vi "Initialize Global Log.vi"(6 "iName":string, 7 "Configuration.Level":T1=enum."Debug", 8 "error in (no error)":errorcluster, 11 "Mediated Actor in":refnum<class "Mediated Actor.lvclass">) -> (0 "error out":errorcluster, 3 "Mediated Actor out":refnum<class "Mediated Actor.lvclass">)   [LabVIEW 2016, in "Stream Mediator.lvlib" / "Mediated Actor.lvclass"]
doc: "--\nCopyright © 2017 Composed SystemsI All rights reserved.\n\nAuthor: Jon McBee <jon.mcbee@composed.io>\n\nThis library is provided \"AS IS\" ,WITHOUT WARRANTIES OR\nCONDITIONS OF ANY KIND, either express or implied.\n\nComposed Systems -- composed.io\n\nStream 0.0.1.1\nJon McBee - Composed Systems\nCopyright (c) 2017, Composed Systems"
uses:
  <userlib>/Composed Systems/Stream/Mediator/Classes/Mediated Actor/Mediated Actor.lvclass
  <userlib>/Composed Systems/Stream/Log/Application Log/Log Level.ctl
  <userlib>/Composed Systems/Stream/Log/Asynchronous Application Log/Asynchronous Application Log.lvclass
  C:/Program Files (x86)/National Instruments/LabVIEW 2016/user.lib/Composed Systems/Stream/Log/Application Log/Application Log.lvclass
  <userlib>/Composed Systems/Stream/Log/Global Application Log/Global Application Log.lvclass
  <userlib>/Composed Systems/Stream/Log/Application Log/Application Log.lvclass
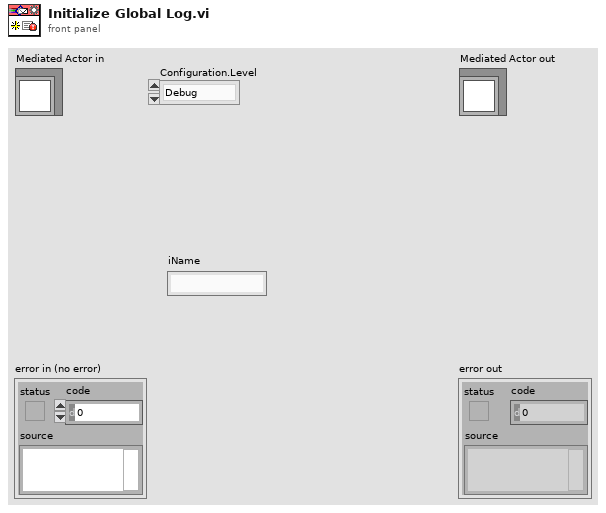
[diagram p1: front panel]
types:
  T1 = typedef "Stream Log.lvlib/Application Log.lvclass/Log Level.ctl" = enum16{"Imperative", "Major", "Minor", "Debug", "Off"}
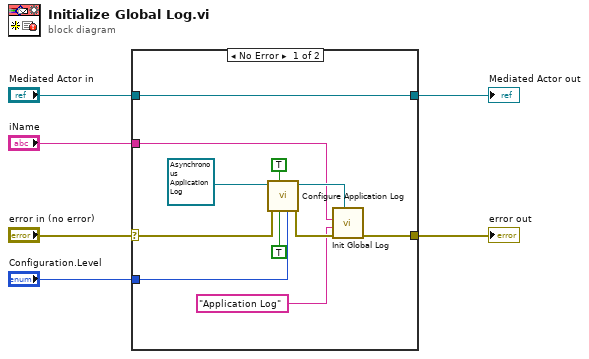
[diagram p0: block diagram]
diagram:
  n1 = case shown="No Error" "error in (no error)" {
    selector: "error in (no error)" -> [w12 w19]
    tunnel: [w10 w19] -> w5
    tunnel: [w17 w18] -> w3
    tunnel: "Mediated Actor in" -> [w17 w18]
    tunnel: "Configuration.Level" -> [w13 _]
    tunnel: "iName" -> [w8 _]
    frame No Error {
      n2 = call-dynamic "Configure Application Log.vi"("Configuration.Level"=w13, "Configuration.Enabled"=TRUE, "Configuration.Call Chain"=TRUE, "error in (no error)"=w12, "Asynchronous Application Log in"=refnum<class "Asynchronous Application Log.lvclass"> refnum ("Log.lvlib:Asynchronous Application Log.lvclass")) -> ("error out"=w11:errorcluster, "Asynchronous Application Log out"=w9:refnum<class "Asynchronous Application Log.lvclass">)  [unwired: 5 in]
      n3 = call <userlib>:"Init Global Log.vi"("Application Log in"=w9, "error in (no error)"=w11, "iType"="Application Log" ("iName"), "iName"=w8) -> ("error out"=w10:errorcluster)  [unwired: 7 in]
    }
    frame Error {
    }
  }
  "error out" <- w5
  "Mediated Actor out" <- w3
